vi "Read Slider Marker Values[].vi"(9 "SlideScale in":refnum<class "SlideScale.lvclass">) -> (3 "SlideScale out":refnum<class "SlideScale.lvclass">, 4 "Marker Values[]":dbl[](array[numeric]))   [LabVIEW 2014, in "Raspberry Pi Compatible Compiler for LabVIEW.lvlib" / "SlideScale.lvclass"]
uses:
  SlideScale.lvclass
  SlideScale.lvclass/SlideScale.ctl
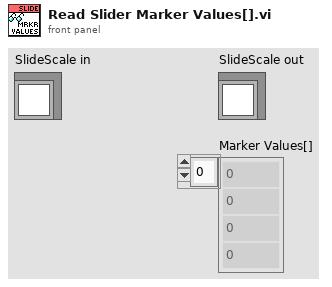
[diagram p1: front panel]
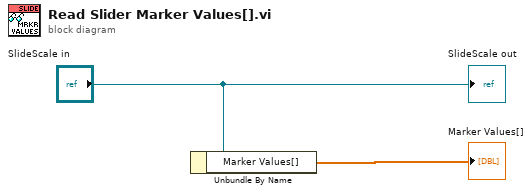
[diagram p0: block diagram]
diagram:
  n1 = Unbundle By Name("SlideScale in") -> ("Marker Values[]"=→"Marker Values[]":dbl[])
  "SlideScale out" <- "SlideScale in"
